vi "Global Lookup.vi"(8 "error in (no error)":errorcluster) -> (0 "error out":errorcluster, 3 "Global Lookup":refnum<data-value>)   [LabVIEW 2019, in "ANODE Tests.lvlib"]
uses:
  ANODE Tests.lvlib
  ANODE/Lookup API/Services/Lookup Service/Lookup Service.lvclass
  ANODE/Lookup API/Providers/Mapped Lookup/Mapped Lookup.lvclass
  C:/Program Files (x86)/National Instruments/LabVIEW 2019/user.lib/ANODE/Lookup API/Services/Lookup Service/Lookup Service.lvclass
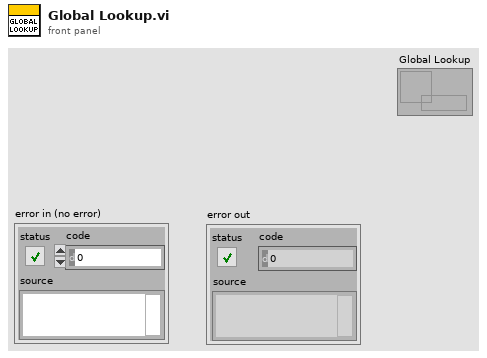
[diagram p1: front panel]
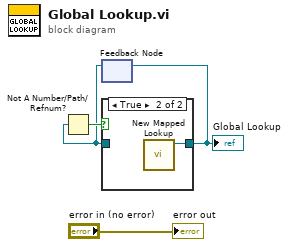
[diagram p0: block diagram]
diagram:
  n1 = feedback #1() -> (w2:refnum<data-value>)  [unwired: 1 in]
  n2 = Not A Number/Path/Refnum?(number/path/refnum=w2) -> (NaN/Path/Refnum?=w3:bool)
  n3 = case shown="True" w3 {
    tunnel: [w5 w6] -> w1
    tunnel: w2 -> [w5 _]
    frame False {
    }
    frame True {
      n4 = call "New Mapped Lookup.vi"() -> ("New Mapped Lookup"=w6:refnum<data-value>)  [unwired: 10 in, 1 out]
    }
  }
  "Global Lookup" <- w1
  n5 = feedback-in #1(w1) -> ()
  "error out" <- "error in (no error)"
